vi "Write Direction.vi"(8 "error in (no error)":errorcluster, 10 "Direction":T1, 11 "Attack in":refnum<class "Net Attack.lvclass">) -> (0 "error out":errorcluster, 3 "Attack out":refnum<class "Net Attack.lvclass">)   [LabVIEW 2014, in "Net Attack.lvclass"]
uses:
  Net Attack.lvclass
  SquareBattle Arena/Direction Enum.ctl
  Net Attack.lvclass/Net Attack.ctl
  SquareBattle Arena/SquareBattle Arena.lvclass
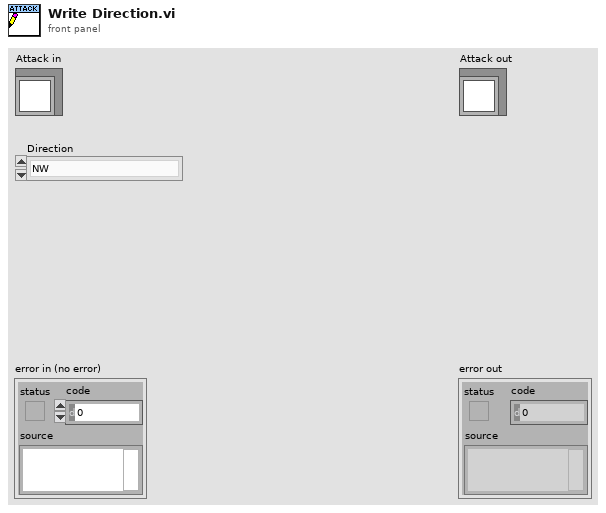
[diagram p1: front panel]
types:
  T1 = typedef "SquareBattle Arena.lvlib/SquareBattle Arena.lvclass/Direction Enum.ctl" = enum16{"NW", "N", "NE", "E", "SE", "S", "SW", "W"}
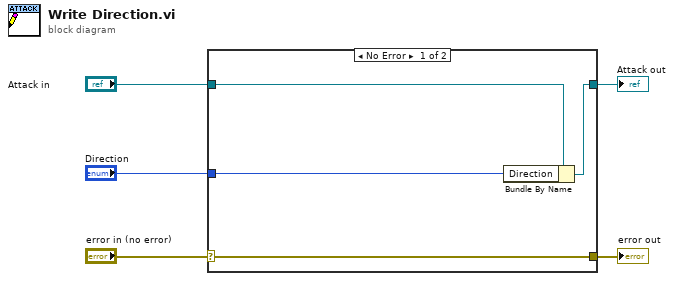
[diagram p0: block diagram]
diagram:
  n1 = case shown="No Error" "error in (no error)" {
    selector: "error in (no error)" -> [w9 w10]
    tunnel: [w9 w10] -> w4
    tunnel: [w7 w11] -> w2
    tunnel: "Attack in" -> [w8 w11]
    tunnel: "Direction" -> [w6 _]
    frame No Error {
      n2 = Bundle By Name(cluster=w8, "Direction"=w6) -> (w7:refnum<class "Net Attack.lvclass">)
    }
    frame Error {
    }
  }
  "error out" <- w4
  "Attack out" <- w2
